vi "LoadCalendarDates.vi"(8 "error in (no error)":errorcluster, 11 "Calendar in":refnum<class "Calendar.lvclass">) -> (0 "error out":errorcluster, 3 "Calendar (dup)":refnum<class "Calendar.lvclass">)   [LabVIEW 2015, in "Calendar.lvclass"]
uses:
  Calendar.lvclass
  <vilib>/Utility/miscctls.llb/LVRowAndColumnTypeDef.ctl
  Calendar.lvclass/Calendar.ctl
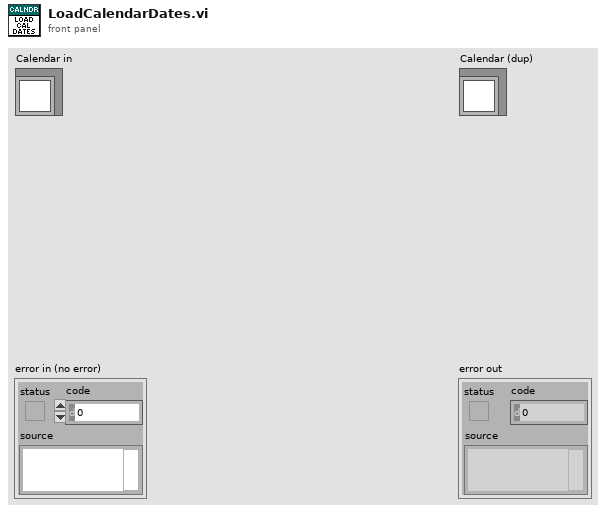
[diagram p1: front panel]
types:
  T1 = typedef "LVRowAndColumnTypeDef.ctl" = cluster{"Row":i32, "Column":i32}
  T2 = typedef "Calendar.lvclass/State Data.ctl" = cluster{"Current Date":timestamp, "First Day of Week":T3, "Color":cluster{"Selector Background":u32, "Selector Text":u32, "Days of Week Background":u32, "Days of Week Text":u32, "Calendar Background":u32, "Calendar Text":u32, "Calendar Selection Background":u32, "Calendar Selection Text":u32}, "Visible":cluster{"Today Selector Visible":bool, "Month-Year Selector Visible":bool}}
  T3 = typedef "Calendar.lvclass/DaysOfWeek.ctl" = enum16{"Sunday", "Monday", "Tuesday", "Wednesday", "Thursday", "Friday", "Saturday"}
  T4 = typedef "LVDateTimeRec.ctl" = cluster{"fractional second":dbl, "second":i32, "minute":i32, "hour":i32, "day of month":i32, "month":i32, "year":i32, "day of week":i32, "day of year":i32, "DST":i32}
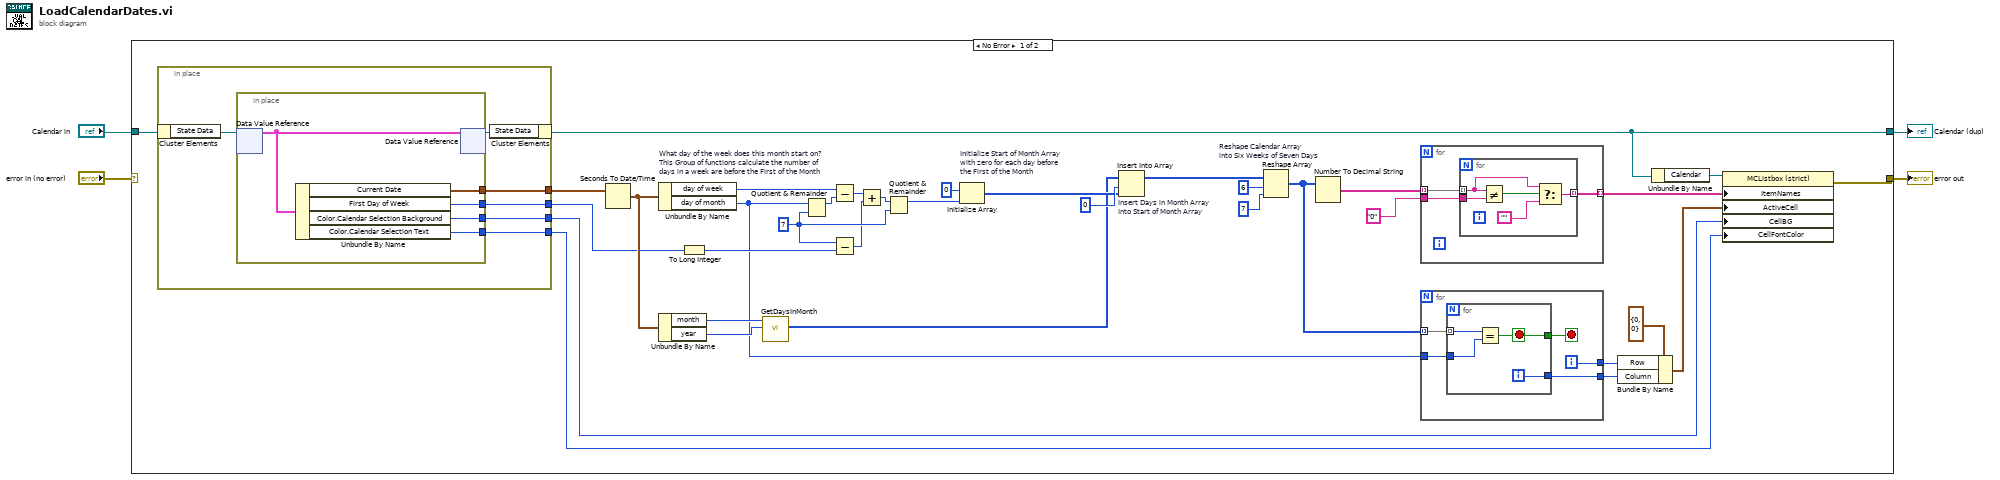
[diagram p0: block diagram]
diagram:
  n1 = case shown="No Error" "error in (no error)" {
    selector: "error in (no error)" -> [_ w69]
    tunnel: [w8 w69] -> w3
    tunnel: [w38 w68] -> w1
    tunnel: "Calendar in" -> [w39 w68]
    frame No Error {
      w37 = 7 ("y")
      n2 = in-place {
        in-place-border: [w61] -> w16
        in-place-border: [w59] -> w11
        in-place-border: [w58] -> w10
        in-place-border: [w57] -> w9
        n3 = in-place-cluster #1(w39) -> ("State Data"=w62:refnum<data-value>)
        n4 = in-place {
          in-place-border: [w66] -> w61
          in-place-border: [w65] -> w59
          in-place-border: [w64] -> w58
          in-place-border: [w63] -> w57
          n5 = in-place-dvr #2(w62) -> (w67:T2)  [unwired: 1 out]
          n6 = Unbundle By Name(w67) -> ("Current Date"=w66:timestamp, "First Day of Week"=w65:T3, "Color.Calendar Selection Background"=w64:u32, "Color.Calendar Selection Text"=w63:u32)
          n7 = in-place-dvr #2(w67) -> (w60:refnum<data-value>)  [unwired: 1 out]
        }
        n8 = in-place-cluster #1("State Data"=w60) -> (w38:refnum<class "Calendar.lvclass">)
      }
      n9 = Seconds To Date/Time(time stamp (now)=w16) -> (date time rec=w23:T4)  [unwired: 1 out]
      n10 = Unbundle By Name "What day of the week does this month start on?\nThis Group of functions calculate the number of\ndays in a week are before the First of the Month"(w23) -> ("day of week"=w26:i32, "day of month"=w18:i32)
      n11 = Unbundle By Name(w23) -> ("month"=w22:i32, "year"=w21:i32)
      n12 = To Long Integer(number=w11) -> (32bit integer=w25:i32)
      n13 = call "GetDaysInMonth.vi"("Year"=w21, "Month"=w22) -> ("Days in Month Array"=w19:i32[])  [unwired: 8 in, 1 out]
      n14 = Quotient & Remainder(x=w18, y=w37) -> (x-y*floor(x/y)=w30:i32)  [unwired: 1 out]
      n15 = Subtract(x=w26, y=w30) -> (x-y=w29:i32)
      n16 = Subtract(x=w37, y=w25) -> (x-y=w28:i32)
      n17 = Add(x=w29, y=w28) -> (x+y=w27:i32)
      n18 = Quotient & Remainder(x=w27, y=w37) -> (x-y*floor(x/y)=w24:i32)  [unwired: 1 out]
      n19 = Initialize Array "Initialize Start of Month Array \nwith zero for each day before \nthe First of the Month"(0, w24) -> (w32:i32[])
      n20 = Insert Into Array "Insert Days in Month Array\nInto Start of Month Array"(array=w19, index=0, new element=w32) -> (w34:i32[])
      n21 = Reshape Array "Reshape Calendar Array\ninto Six Weeks of Seven Days"(w34, 6 ("dimension size"), 7 ("dimension size")) -> (w17:i32[][])
      n22 = Number To Decimal String(number=w17) -> (decimal integer string=w7:string[][])  [unwired: 1 in]
      n23 = for {
        tunnel: w7 -> [w42] mode=indexing
        tunnel: "0" -> [w41]
        tunnel: [w40] -> w5 mode=indexing
        n24 = for {
          tunnel: w42 -> [w45] mode=indexing
          tunnel: w41 -> [w47]
          tunnel: [w43] -> w40 mode=indexing
          n25 = Not Equal?(x=w45, y=w47) -> (x != y?=w46:bool)
          n26 = Select(t=w45, s=w46, f="") -> (s? t:f=w43:string)
        }
      }
      n27 = for {
        tunnel: w18 -> [w51]
        tunnel: w17 -> [w52] mode=indexing
        tunnel: [w49] -> w14
        tunnel: [w48] -> w13
        i -> [w49]
        stop <- w50 stop-if-true
        n28 = for {
          tunnel: w52 -> [w56] mode=indexing
          tunnel: w51 -> [w55]
          tunnel: [w54] -> w50
          tunnel: [w53] -> w48
          i -> [w53]
          stop <- w54 stop-if-true
          n29 = Equal?(x=w56, y=w55) -> (x = y?=w54:bool)
        }
      }
      n30 = Bundle By Name(cluster=T1 {"Row"=0, "Column"=0} ("Active Cell:Active Cell"), "Row"=w14, "Column"=w13) -> (w12:T1)
      n31 = Unbundle By Name(w38) -> ("Calendar"=w20:refnum<vi>)
      n32 = property class="MCListbox (strict)"(reference=w20, "ItemNames"=w5, "ActiveCell"=w12, "CellBG"=w10, "CellFontColor"=w9) -> (error out=w8:errorcluster)  [unwired: 1 in, 1 out]
    }
    frame Error {
    }
  }
  "error out" <- w3
  "Calendar (dup)" <- w1
